vi "umToslm.vi"(1 "X (um)":dbl) -> (0 "SLM Period":dbl)   [LabVIEW 2020]
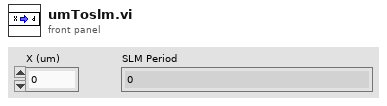
[diagram p1: front panel]
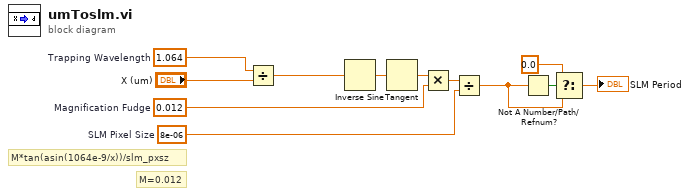
[diagram p0: block diagram]
diagram:
  w9 = 8e-06  # SLM Pixel Size
  w10 = 0.012  # Magnification Fudge
  w11 = 1.064  # Trapping Wavelength
  # "M=0.012"
  # "M*tan(asin(1064e-9/x))/slm_pxsz"
  n1 = Divide(x=w11, y="X (um)") -> (x/y=w6:dbl)
  n2 = Inverse Sine(1:w6) -> (0:w7:dbl)
  n3 = Tangent(1:w7) -> (0:w5:dbl)
  n4 = Multiply(x=w5, y=w10) -> (x*y=w8:dbl)
  n5 = Divide(x=w8, y=w9) -> (x/y=w3:dbl)
  n6 = Not A Number/Path/Refnum?(number/path/refnum=w3) -> (NaN/Path/Refnum?=w4:bool)
  n7 = Select(t=0.0, s=w4, f=w3) -> (s? t:f=→"SLM Period":dbl)
